vi "Pressure Device (Read).vi"(6 "ISOBUS address":T9=-1 caption="ISOBUS address (-1)", 8 "error in":errorcluster, 11 "Mercury Reference In":T10) -> (0 "error out":errorcluster, 2 "Device Details":T2, 3 "Mercury Reference Out":T10, 4 "Valid?":T1)   [LabVIEW 2018, in "Mercury iXX.lvlib" / "Pressure.lvlib"]
doc: "Read the current device configuration for the selected pressure device."
uses:
  Pressure.lvlib
  Mercury Reference.ctl
  Comms Transport Layer.ctl
  Query Dynamic Reference.ctl
  ISOBus Address.ctl
  Pressure Device (Read).ctl
  Manufacturing Data.ctl
  Pressure Sensor Type.ctl
  Mercury iXX.lvlib_Pressure/Calibration Cluster.ctl
  Mercury iXX.lvlib_Pressure/Calibration Interpolation.ctl
  Mercury iXX.lvlib_Pressure/Loop Cluster.ctl
  Pressure Signals Cluster.ctl
  Is Valid LED.ctl
  Command Verbs.ctl
  Mercury iXX.lvlib
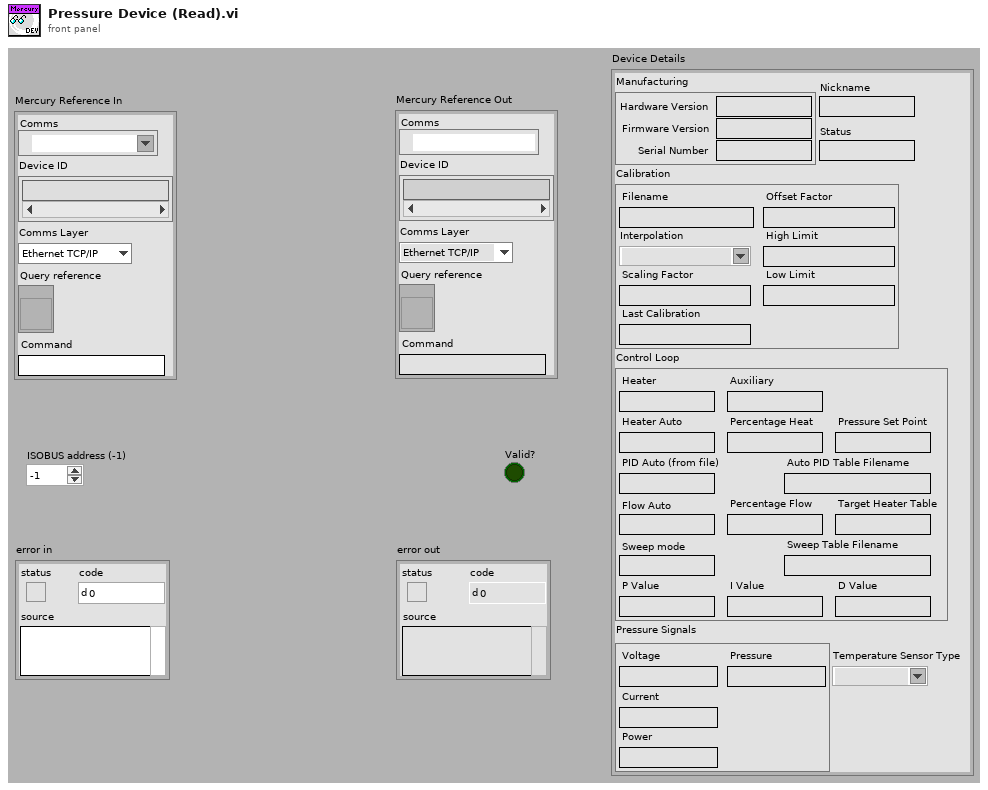
[diagram p1: front panel]
types:
  T1 = typedef "Mercury iXX.lvlib/Is Valid LED.ctl" = bool
  T2 = typedef "Mercury iXX.lvlib/Pressure.lvlib/Pressure Device (Read).ctl" = cluster{"Manufacturing":T3, "Temperature Sensor Type":T4, "Calibration":T5, "Control Loop":T7, "Pressure Signals":T8, "Nickname":string, "Status":string}
  T3 = typedef "Mercury iXX.lvlib/Manufacturing Data.ctl" = cluster{"Hardware Version":string, "Firmware Version":string, "Serial Number":string}
  T4 = typedef "Mercury iXX.lvlib/Pressure.lvlib/Pressure Sensor Type.ctl" = string
  T5 = typedef "Mercury iXX.lvlib/Pressure.lvlib/Calibration Cluster.ctl" = cluster{"Filename":string, "Interpolation":T6, "Scaling Factor":string, "Offset Factor":string, "High Limit":string, "Low Limit":string, "Last Calibration":string}
  T6 = typedef "Mercury iXX.lvlib/Pressure.lvlib/Calibration Interpolation.ctl" = string
  T7 = typedef "Mercury iXX.lvlib/Pressure.lvlib/Loop Cluster.ctl" = cluster{"Heater":string, "Auxiliary":string, "Heater Auto":string, "Percentage Heat":string, "Pressure Set Point":string, "PID Auto (from file)":string, "P Value":string, "I Value":string, "D Value":string, "Auto PID Table Filename":string, "Flow Auto":string, "Target Heater Table":string, "Sweep mode":string, "Sweep Table Filename":string, "Percentage Flow":string}
  T8 = typedef "Mercury iXX.lvlib/Pressure.lvlib/Pressure Signals Cluster.ctl" = cluster{"Voltage":string, "Current":string, "Power":string, "Pressure":string}
  T9 = typedef "Mercury iXX.lvlib/ISOBus Address.ctl" = i32
  T10 = typedef "Mercury iXX.lvlib/Mercury Reference.ctl" = cluster{"Comms":refnum<visa-resource-name>, "Device ID":string[], "Comms Layer":T11, "Command":string, "Query reference":T12}
  T11 = typedef "Mercury iXX.lvlib/Comms Transport Layer.ctl" = enum16{"Ethernet TCP/IP", "USB", "ISOBus - RS-232", "GPIB"}
  T12 = typedef "Mercury iXX.lvlib/Query Dynamic Reference.ctl" = refnum<vi>
  T13 = typedef "Mercury iXX.lvlib/Command Verbs.ctl" = string
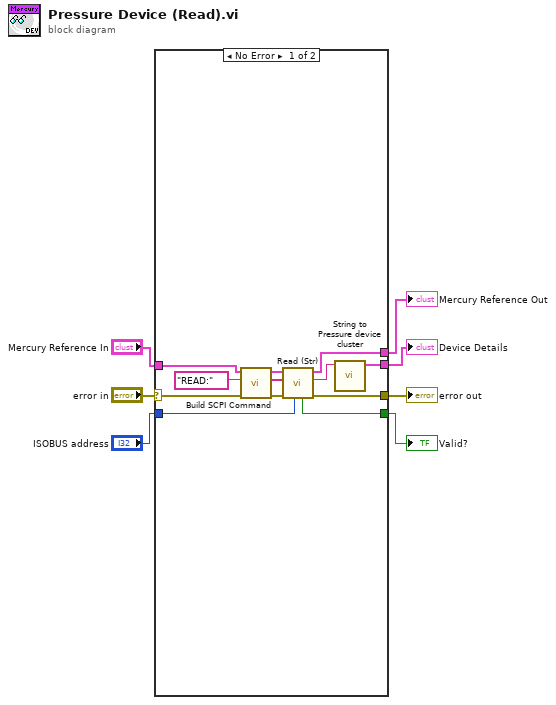
[diagram p0: block diagram]
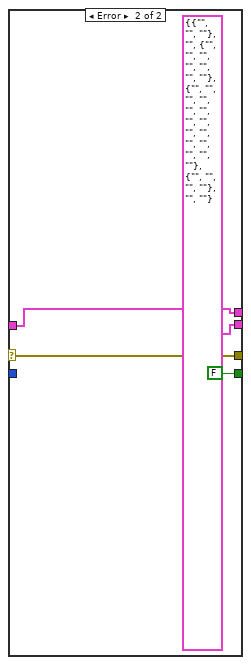
[diagram p2: hidden frame]
diagram:
  n1 = case shown="No Error" "error in" {
    selector: "error in" -> [w8 w23]
    tunnel: "Mercury Reference In" -> [w13 w21]
    tunnel: [w11 w23] -> w6
    tunnel: [w12 w21] -> w5
    tunnel: "ISOBUS address" -> [w9 _]
    tunnel: [w10 T1 FALSE ("Valid?")] -> w3
    tunnel: [w19 T2 {"Manufacturing"={"Hardware Version"="", "Firmware Version"="", "Serial Number"=""}, "Temperature Sensor Type"="", "Calibration"={"Filename"="", "Interpolation"="", "Scaling Factor"="", "Offset Factor"="", "High Limit"="", "Low Limit"="", "Last Calibration"=""}, "Control Loop"={"Heater"="", "Auxiliary"="", "Heater Auto"="", "Percentage Heat"="", "Pressure Set Point"="", "PID Auto (from file)"="", "P Value"="", "I Value"="", "D Value"="", "Auto PID Table Filename"="", "Flow Auto"="", "Target Heater Table"="", "Sweep mode"="", "Sweep Table Filename"="", "Percentage Flow"=""}, "Pressure Signals"={"Voltage"="", "Current"="", "Power"="", "Pressure"=""}, "Nickname"="", "Status"=""} ("Temperature Device Settings")] -> w2
    frame No Error {
      n2 = call "Build SCPI Command.vi"("error in"=w8, "Verb"=T13 "READ:", "Mercury Reference In"=w13) -> ("error out"=w18:errorcluster, "SCPI Message(s)"=w15:string[], "Mercury Reference Out"=w16:T10)  [unwired: 1 in, 5 out]
      n3 = call "Read (Str).vi"("ISOBUS address"=w9, "error in"=w18, "SCPI Message(s)"=w15, "Mercury Reference In"=w16) -> ("error out"=w11:errorcluster, "Response"=w14:string, "Mercury Reference Out"=w12:T10, "Valid?"=w10:T1)  [unwired: 4 out]
      n4 = call "String to Pressure device cluster.vi"("Pressure Device Details"=w14) -> ("Pressure Device Settings"=w19:T2)  [unwired: 1 in, 9 out]
    }
    frame Error {
    }
  }
  "Mercury Reference Out" <- w5
  "error out" <- w6
  "Device Details" <- w2
  "Valid?" <- w3
